vi "TEST_L0_DELAYLINES_(1ST)_NEW.vi"(7 "Serial Number":string="SN_00187", 8 "error in (no error)":errorcluster, 11 "Instrument VISA in":T1={"AWG VISA"="AgilentGen1", "Oscilloscope  VISA "="AgilentOsc", "Integration Board IP"="172.16.17.47", "connection ID"=refnum, "report out"=refnum, "report file path"=path "C:/Users/omartinez/Desktop/L0nL1_Results"}) -> (0 "error out":errorcluster, 3 "Instrument VISA out":T1={"AWG VISA"="AgilentGen1", "Oscilloscope  VISA "="AgilentOsc", "Integration Board IP"="172.16.17.47", "connection ID"=refnum, "report out"=refnum, "report file path"=path "C:/Users/omartinez/Desktop/L0nL1_Results"})   [LabVIEW 2012]
uses:
  <vilib>/Utility/NIReport.llb/NI_report.lvclass
  <vilib>/Utility/NIReport.llb/HTML/NI_HTML.lvclass
  <instrlib>/Agilent 8000 Series/Public/Configure/Configure Math (Binary Operation).vi
  Sum_Abrilader/L0_Sum_Adder Folder/C/Program Files/National Instruments/LabVIEW 2012/instr.lib/Agilent 8000 Series/Public/Data/Low Level/Fetch Measurement (More).vi
  <instrlib>/Agilent 8000 Series/Public/Data/Read Measurement (More).vi
  <instrlib>/Agilent 8000 Series/Agilent 8000 Series.lvlib
panel:
  out "Measured Delay":dbl=-8.19193e-09 caption="Measurement"
  in  "Input Voltage":dbl=0.5
  in  "Channels":i32[](array[numeric])=[0, 1, 2, 3, 4, 5, 6]
  in  "Amp Scaler":dbl=0.5
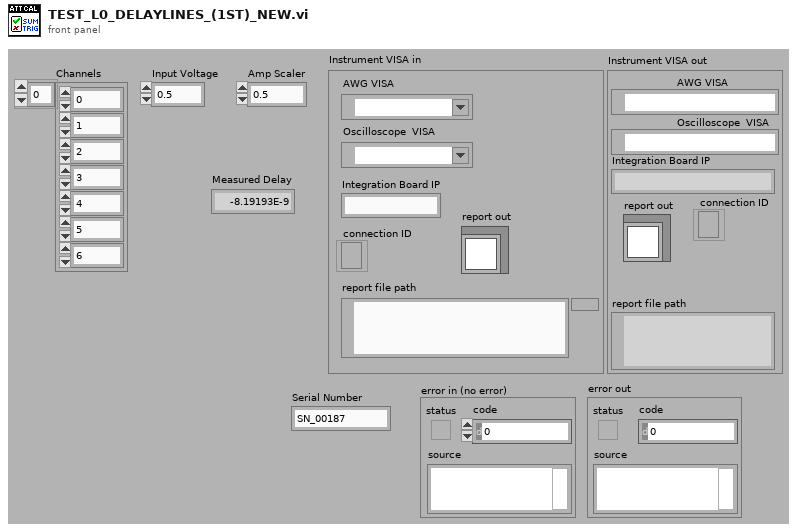
[diagram p1: front panel]
types:
  T1 = cluster{"AWG VISA":refnum<visa-resource-name>, "Oscilloscope  VISA ":refnum<visa-resource-name>, "Integration Board IP":string, "connection ID":refnum<k5>, "report out":refnum<class "NI_report.lvclass">, "report file path":path}
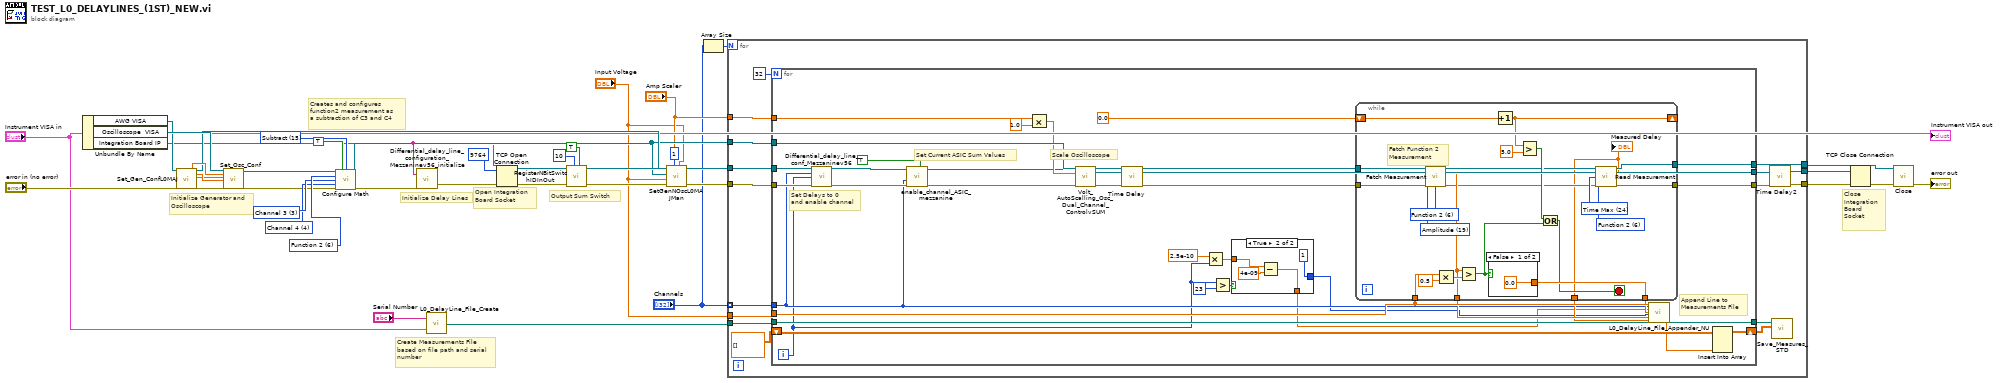
[diagram p0: block diagram]
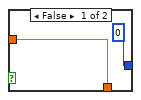
[diagram p2: hidden frame]
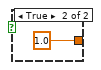
[diagram p3: hidden frame]
diagram:
  w20 = u16 6 items=["Function 1"=5, "Function 2"=6, "Function 3"=7, "Function 4"=8] ("Math Channel (5: Function 1)")
  w21 = u16 15 items=["Add"=12, "Divide"=13, "Multiply"=14, "Subtract"=15, "Common Mode"=16, "Versus"=17] ("Math Operation (12: Add)")
  w19 = 3 items=["Channel 1"=1, "Channel 2"=2, "Channel 3"=3, "Channel 4"=4] ("Channel (1: Channel 1)")
  w18 = 4 items=["Channel 1"=1, "Channel 2"=2, "Channel 3"=3, "Channel 4"=4] ("Channel (1: Channel 1)")
  # "Create Measurements File\nbased on file path and serial\nnumber"
  # "Close \nIntegration \nBoard \nSocket"
  # "Output Sum Switch"
  # "Open Integration\nBoard Socket"
  # "Initialize Delay Lines"
  # "Initialize Generator and \nOscilloscope"
  # "Creates and configures\nfunction2 measurement as\na subtraction of C3 and C4"
  n1 = Unbundle By Name("Instrument VISA in") -> ("AWG VISA"=w37:refnum<visa-resource-name>, "Oscilloscope  VISA"=w38:refnum<visa-resource-name>, "Integration Board IP"=w10:string)
  n2 = call "Set_Gen_ConfL0MAJ.vi"("AWG VISA"=w37, "error in (no error)"="error in (no error)") -> ("Amplitude 1 OUT"=w35:dbl, "VISA resource name out"=w29:refnum<visa-resource-name>, "Pulse Width in seconds 1 OUT"=w34:dbl, "Trigger Level 1"=w33:dbl, "error out"=w39:errorcluster)  [unwired: 10 in, 3 out]
  n3 = call "Set_Osc_Conf.vi"("VISA resource name"=w38, "Amplitude IN"=w35, "Trigger Level IN"=w33, "Pulse Width in seconds IN"=w34, "error in (no error)"=w39) -> ("VISA resource name out"=w17:refnum<visa-resource-name>, "error out"=w16:errorcluster)  [unwired: 13 in]
  n4 = call-poly <instrlib>:"Configure Math.vi"("VISA resource name"=w17, "Enable Math Channel (T:Enable)"=TRUE, "Math Operation (12: Add)"=w21, "Math Channel (5: Function 1)"=w20, "Math Operand (1: Channel 1)"=w19, "Math Operand (2: Channel 2)"=w18, "error in (no error)"=w16) -> ("VISA resource name out"=w14:refnum<visa-resource-name>, "error out"=w15:errorcluster)  [unwired: 7 in]
  n5 = call "Differential_delay_line_configuration_Mezzaninev56_initialize.vi"("error in (no error)"=w15, "address"=w10) -> ("error out 2"=w32:errorcluster)
  n6 = call "L0_DelayLine_File_Create.vi"("input cluster"="Instrument VISA in", "Serial Number"="Serial Number") -> ("appended path"=w11:path)
  n7 = TCP Open Connection(address=w10, remote port or service name=9764, error in (no error)=w32) -> (connection ID=w27:refnum<k5>, error out=w31:errorcluster)  [unwired: 2 in]
  n8 = call "RegisterNBitSwitchIDInOut.vi"("Switch Bit"=TRUE, "N Bit"=10, "error in (no error)"=w31, "connection ID"=w27) -> ("error out"=w28:errorcluster, "connection ID out"=w26:refnum<k5>)  [unwired: 5 in]
  n9 = call "SetGenNOscL0MAJMan.vi"("Input Voltage"="Input Voltage", "Amp Scaler"="Amp Scaler", "NChannels"=1, "error in (no error)"=w28, "Output Voltage"="Input Voltage", "VISA resource name"=w14, "AWG VISA"=w29) -> ("error out 2"=w9:errorcluster)  [unwired: 4 in]
  n10 = Array Size(array="Channels") -> (size(s)=w6:i32)
  n11 = for {
    N: w6 -> [_]
    tunnel: [w43] -> w30
    tunnel: w26 -> [w55]
    tunnel: [w54] -> w23
    tunnel: w14 -> [w53]
    tunnel: w11 -> [w52]
    tunnel: w9 -> [w51]
    tunnel: "Amp Scaler" -> [w50]
    tunnel: "Channels" -> [w49] mode=indexing
    tunnel: "Input Voltage" -> [w48]
    tunnel: [w41] -> w1
    n12 = for {
      N: 32 -> [_]
      tunnel: [w89] -> w42
      tunnel: w55 -> [w88]
      tunnel: [w75] -> w54
      tunnel: w53 -> [w87]
      tunnel: w52 -> [w86]
      tunnel: w51 -> [w85]
      tunnel: w50 -> [w84]
      tunnel: w49 -> [w63]
      tunnel: w48 -> [w74]
      shift-right: [w69] -> w45
      shift-left: dbl[][] [] ("Y") -> [w71]
      tunnel: [w68] -> w44
      tunnel: [w65] -> w41
      i -> [w61]
      # "Scale Oscilloscope"
      # "Set Current ASIC Sum Values"
      # "Append Line to \nMeasurements File"
      # "Set Delays to 0 \nand enable channel"
      n13 = call "Differential_delay_line_conf_Mezzaninev56.vi"("connection ID"=w88, "channel"=w63, "Delay value"=w61, "error in (no error)"=w85) -> ("connection ID out"=w82:refnum<k5>, "error out 2"=w83:errorcluster)  [unwired: 4 in, 6 out]
      n14 = call "enable_channel_ASIC_mezzanine.vi"("maj/sum"=TRUE, "error in"=w83, "Channel"=w63, "connection ID"=w82) -> ("error out"=w76:errorcluster, "connection ID out"=w75:refnum<k5>)  [unwired: 5 in, 1 out]
      n15 = Multiply(x=w84, y=1.0) -> (x*y=w78:dbl)
      n16 = call "Volt_AutoScalling_Osc_Dual_Channel_ControlvSUM.vi"("VISA Oscilloscope"=w87, "Voltage In"=w78, "error in"=w76) -> ("VISA resource name out"=w79:refnum<visa-resource-name>, "error out"=w80:errorcluster)  [unwired: 11 in]
      n17 = call "Time Delay"("error in (no error)"=w80) -> ("error out"=w66:errorcluster)  [unwired: 10 in]
      n18 = Multiply(x=2.5e-10, y=w61) -> (x*y=w57:dbl)
      n19 = Greater?(x=w61, y=23) -> (0:w59:bool)
      n20 = case shown="True" w59 {
        tunnel: [0 ("y") 1 ("y")] -> w58
        tunnel: w57 -> [w90 w93]
        tunnel: [w90 w94] -> w56
        frame False {
        }
        frame True {
          n21 = Subtract(x=w93, y=4e-09) -> (x-y=w94:dbl)
        }
      }
      n22 = while {
        tunnel: [w99] -> w89
        tunnel: w66 -> [w115]
        tunnel: w79 -> [w114]
        tunnel: w74 -> [w112]
        tunnel: [w110] -> w73
        tunnel: [w109] -> w72
        shift-right: [w107] -> _
        shift-left: 0.0 ("Status") -> [w108]
        tunnel: [w97] -> w65
        tunnel: [w96] -> w64
        stop <- w103 stop-if-true
        w101 = 6 items=["Channel 1"=1, "Channel 2"=2, "Channel 3"=3, "Channel 4"=4, "Function 1"=5, "Function 2"=6, "Function 3"=7, "Function 4"=8, "Memory 1"=9, "Memory 2"=10, "Memory 3"=11, "Memory 4"=12] ("Channel (1: Channel 1)")
        w102 = 24 items=["Rise Time", "Fall Time", "Frequency", "Period", "Voltage RMS(AC)", "Voltage RMS(DC)", "Voltage RMS (AC,cycle)", "Voltage RMS (DC,cycle)", "Voltage Max", "Voltage Min", "Voltage Middle", "Voltage Vpp", "Voltage High", "Voltage Low", "Voltage Average", "Voltage Average (cycle)", "Width Negative", "Width Positive", "Duty Cycle Positive", "Amplitude", "Overshoot", "Preshoot", "Voltage Base", "Voltage Upper", "Time Max", "Time Min", "Color Grade Crossing", "Color Grade Eye Width", "Color Grade Eye Height", "Color Grade Eye Q-Factory", "Color Grade Eye Duty Cycle Distortion(Percent)", "Color Grade Eye Duty Cycle Distortion(Time)", "Color Grade Eye Jitter(PP)", "Color Grade Eye Width(RMS)", "Cycle-cycle Duty Jitter(Rising)", "Cycle-cycle Duty Jitter(Falling)", "Cycle-cycle Jitter(Rising)", "Cycle-cycle Jitter(Falling)", "Cycle-cycle - Width", "Cycle-cycle + Width", "Date Rate", "Unit Interval", "FFT Delta Frequency", "FFT Delta Magnitude", "FFT Frequency", "FFT Magnitude", "Slew Rate", "Area (Entire Display)", "Area(Single Cycle)", "Duty Cycle (Rising)", "Duty Cycle (Falling)"] ("Measurement Function (0: Rise Time)")
        w117 = 19 items=["Rise Time", "Fall Time", "Frequency", "Period", "Voltage RMS(AC)", "Voltage RMS(DC)", "Voltage RMS (AC,cycle)", "Voltage RMS (DC,cycle)", "Voltage Max", "Voltage Min", "Voltage Middle", "Voltage Vpp", "Voltage High", "Voltage Low", "Voltage Average", "Voltage Average (cycle)", "Width Negative", "Width Positive", "Duty Cycle Positive", "Amplitude", "Overshoot", "Preshoot", "Voltage Base", "Voltage Upper", "Time Max", "Time Min", "Color Grade Crossing", "Color Grade Eye Width", "Color Grade Eye Height", "Color Grade Eye Q-Factory", "Color Grade Eye Duty Cycle Distortion(Percent)", "Color Grade Eye Duty Cycle Distortion(Time)", "Color Grade Eye Jitter(PP)", "Color Grade Eye Width(RMS)", "Cycle-cycle Duty Jitter(Rising)", "Cycle-cycle Duty Jitter(Falling)", "Cycle-cycle Jitter(Rising)", "Cycle-cycle Jitter(Falling)", "Cycle-cycle - Width", "Cycle-cycle + Width", "Date Rate", "Unit Interval", "FFT Delta Frequency", "FFT Delta Magnitude", "FFT Frequency", "FFT Magnitude", "Slew Rate", "Area (Entire Display)", "Area(Single Cycle)", "Duty Cycle (Rising)", "Duty Cycle (Falling)"] ("Measurement Function (0: Rise Time)")
        w116 = 6 items=["Channel 1"=1, "Channel 2"=2, "Channel 3"=3, "Channel 4"=4, "Function 1"=5, "Function 2"=6, "Function 3"=7, "Function 4"=8, "Memory 1"=9, "Memory 2"=10, "Memory 3"=11, "Memory 4"=12] ("Channel (1: Channel 1)")
        # "Fetch Function 2\nMeasurement"
        n23 = call-poly "Fetch Measurement.vi"("VISA resource name"=w114, "Channel (1: Channel 1)"=w116, "Measurement Function (0: Rise Time)"=w117, "error in (no error)"=w115) -> ("VISA resource name out"=w98:refnum<visa-resource-name>, "Measurement"=w109:dbl, "error out"=w100:errorcluster)  [unwired: 9 in]
        n24 = Multiply(x=w112, y=0.5) -> (x*y=w113:dbl)
        n25 = Greater?(x=w109, y=w113) -> (0:w104:bool)
        n26 = case shown="False" w104 {
          tunnel: [0.0 ("Status") 1.0 ("Status")] -> w110
          frame False {
          }
          frame True {
          }
        }
        n27 = Increment(x=w108) -> (x+1=w107:dbl)
        n28 = Greater?(x=w107, y=5.0) -> (0:w105:bool)
        n29 = Or(x=w105, y=w104) -> (x .or. y?=w103:bool)
        n30 = call-poly <instrlib>:"Read Measurement.vi"("VISA resource name"=w98, "Channel (1: Channel 1)"=w101, "Measurement Function (0: Rise Time)"=w102, "error in (no error)"=w100) -> ("VISA resource name out"=w97:refnum<visa-resource-name>, "Measurement"=w96:dbl, "error out"=w99:errorcluster)  [unwired: 9 in]
        "Measured Delay" <- w96
      }
      n31 = call "L0_DelayLine_File_Appender_NU.vi"("Vin"=w74, "CH"=w63, "DelayLine"=w56, "Status"=w73, "Path"=w58, "Vmeas"=w72, "Measured Delay"=w64, "file path (dialog if empty)"=w86) -> ("appended array"=w70:dbl[], "file path (dialog if empty) 2"=w68:path)  [unwired: 18 in]
      n32 = Insert Into Array(array=w71, new element=w70) -> (w69:dbl[][])  [unwired: 2 in]
    }
    n33 = call "Time Delay2"("error in (no error)"=w42) -> ("error out"=w43:errorcluster)  [unwired: 10 in]
    n34 = call "Save_Measures_STD.vi"("Data in"=w45, "file path (dialog if empty)"=w44) -> ()  [unwired: 10 in]
  }
  n35 = TCP Close Connection(connection ID=w23, error in (no error)=w30) -> (error out=w3:errorcluster)  [unwired: 1 in, 1 out]
  n36 = call <instrlib>:"Close.vi"("error in (no error)"=w3, "VISA resource name"=w1) -> ("error out"=→"error out":errorcluster)  [unwired: 9 in]
  "Instrument VISA out" <- "Instrument VISA in"
